vi "RSNRPZ Get Time Slot Mid Offset.vi"(8 "error in (no error)":errorcluster, 10 "Channel (1)":i32=1, 11 "VISA session":refnum<visa-resource-name> caption="VISA resource name") -> (0 "error out":errorcluster, 2 "Offset":dbl format="%^.3e", 3 "dup VISA session":refnum<visa-resource-name> caption="VISA resource name")   [LabVIEW 2010]
doc: "This VI queries the start of an exclusion interval in a timeslot.\n\nRemote-control command(s):\nSENSe:POWer:TSLot[:AVG]:MID:OFFSet?"
uses:
  rsnrpz_32.dll
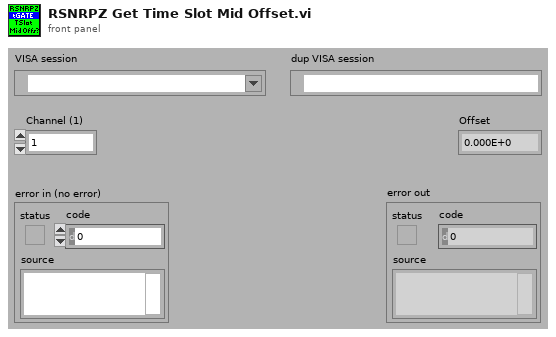
[diagram p1: front panel]
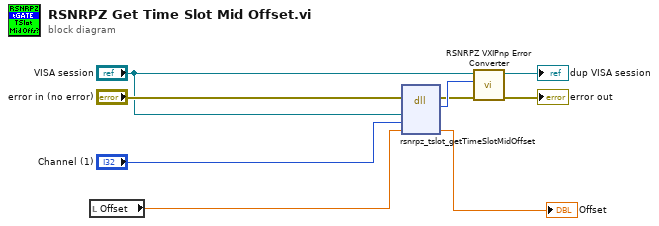
[diagram p0: block diagram]
diagram:
  n1 = local read "Offset"() -> (w7:dbl)
  n2 = dll-call lib="rsnrpz_32.dll" fn="rsnrpz_tslot_getTimeSlotMidOffset"(error in="error in (no error)", "Instrument Handle"="VISA session", "Channel"="Channel (1)", "Offset"=w7) -> (error out=w5:errorcluster, "Status"=w9:i32, "Offset"=→"Offset":dbl)  [unwired: 4 in, 1 out]
  n3 = call <instrlib>:"RSNRPZ VXIPnp Error Converter.vi"("error in"=w5, "VXIPnp error code"=w9, "VISA session"="VISA session") -> ("error out"=→"error out":errorcluster, "dup VISA session"=→"dup VISA session":refnum<visa-resource-name>)  [unwired: 7 in]
